vi "Write Key DBL.vi"(6 "Insert If Not Exist(T)":bool=TRUE, 7 "Section Name":string, 8 "error in (no error)":errorcluster, 9 "Key Value":dbl, 10 "Key Name":string, 11 "Config Data":T1(array[cluster])=[{"Section Name"="General", "Section Data"=[["MatchSeqFile", "Hi6825RLIV100D.seq"], ["CorrOffsetFilePath", ""]]}, {"Section Name"="PluginCfg", "Section Data"=[]}, {"Section Name"="CompCfg", "Section Data"=[["Index", "TestName", "TestNumber", "NormVal", "Units", "Checked", "LowLimit", "HighLimit", "KUG_1"], ["1", "RF_Gain_ChA_HG_35001", "3", "0", "dBm", "T", "0", "0", "0"], ["2", "RF_Gain_ChB_HG_3500", "4", "0", "dBm", "T", "0", "0", "0"], ["3", "RF_NF_ChA_LG_3500", "5", "0", "", "T", "0", "0", "0"], ["4", "RF_NF_ChB_LG_3500", "6", "0", "", "T", "0", "0", "0"], ["5", "RF_NF_ChA_HG_3500", "7", "0", "", "T", "0", "0", "0"], ["6", "RF_NF_ChB_HG_3500", "8", "0", "", "T", "0", "0", "0"], ["7", "RF_InsertionLoss_ChA_3500", "9", "0", "dBm", "T", "0", "0", "0"], ["8", "RF_InsertionLoss_ChB_3500", "10", "0", "dBm", "T", "0", "0", "0"], ["9", "RF_InsertionLoss_CHA_FixedFreq_100", "11", "0", "dBm", "T", "0", "0", "0"], ["10", "RF_InsertionLoss_CHB_FixedFreq_100", "12", "0", "dBm", "T", "0", "0", "0"], ["11", "RF_Gain_ChA_HG_3500", "113", "0", "dBm", "T", "0", "0", "0"], ["12", "RF_Gain_ChB_HG_3500", "114", "0", "dBm", "T", "0", "0", "0"], ["13", "RF_NF_ChA_LG_3500", "115", "0", "", "T", "0", "0", "0"], ["14", "RF_NF_ChB_LG_3500", "116", "0", "", "T", "0", "0", "0"], ["15", "RF_NF_ChA_HG_3500", "117", "0", "", "T", "0", "0", "0"], ["16", "RF_NF_ChB_HG_3500", "118", "0", "", "T", "0", "0", "0"], ["17", "RF_InsertionLoss_ChA_3500", "119", "0", "dBm", "T", "0", "0", "0"], ["18", "RF_InsertionLoss_ChB_3500", "120", "0", "dBm", "T", "0", "0", "0"], ["19", "RF_InsertionLoss_CHA_FixedFreq_100", "121", "0", "dBm", "T", "0", "0", "0"], ["20", "RF_InsertionLoss_CHB_FixedFreq_100", "122", "0", "dBm", "T", "0", "0", "0"]]}]) -> (0 "error out":errorcluster, 3 "Config Data dup":T1(array[cluster]))   [LabVIEW 2020, in "GUCalibration2.lvlib"]
uses:
  GUCalibration2.lvlib
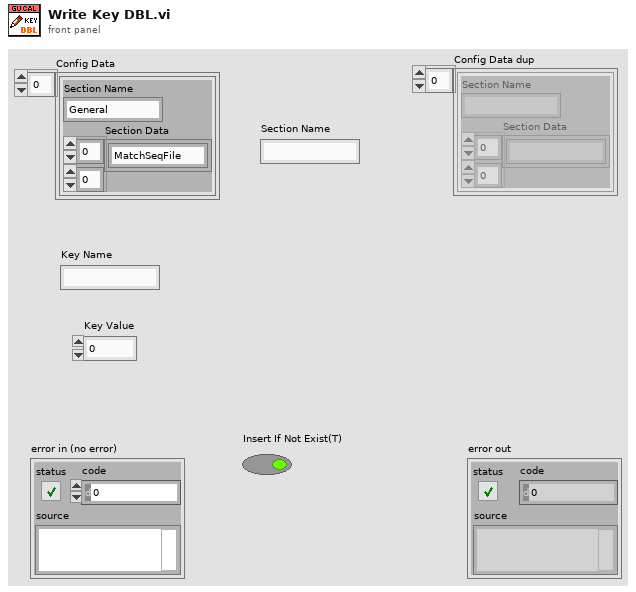
[diagram p1: front panel]
types:
  T1 = cluster{"Section Name":string, "Section Data":string[][]}[]
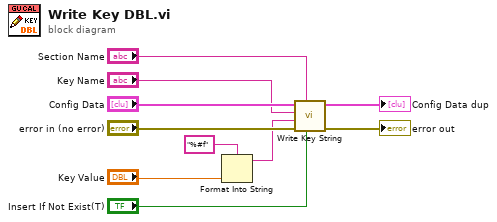
[diagram p0: block diagram]
diagram:
  n1 = Format Into String(format string="%#f", "Key Value") -> (resulting string=w1:string)  [unwired: 2 in, 1 out]
  n2 = call "Write Key String.vi"("Insert If Not Exist(T)"="Insert If Not Exist(T)", "Section Name"="Section Name", "error in (no error)"="error in (no error)", "Key Value"=w1, "Key Name"="Key Name", "Config Data"="Config Data") -> ("error out"=→"error out":errorcluster, "Config Data dup"=→"Config Data dup":T1)  [unwired: 4 in]
